vi "delete control from class private data.vi"(8 "error in":errorcluster, 9 "control label":string, 10 "path":path, 11 "Project in":refnum<vi>) -> (0 "error out":errorcluster, 3 "Project out":refnum<vi>)   [LabVIEW 2013, in "NISE Tools Scripting.lvlib"]
uses:
  NISE Tools Scripting.lvlib
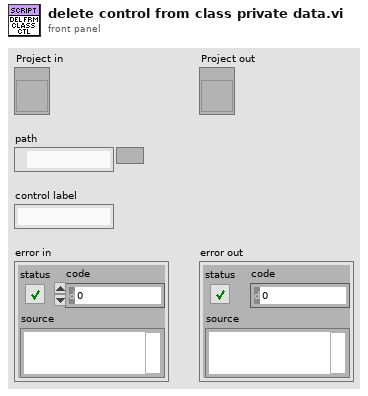
[diagram p1: front panel]
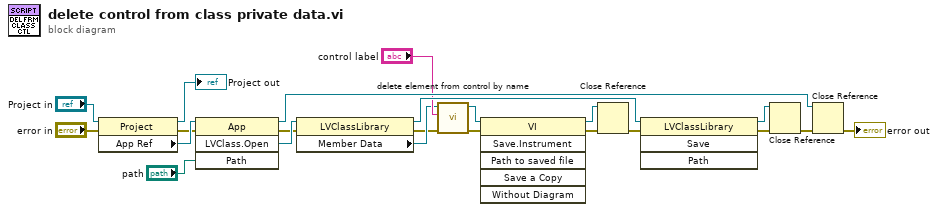
[diagram p0: block diagram]
diagram:
  n1 = property class="Project"(reference="Project in", error in="error in") -> (reference out=→"Project out":refnum<vi>, error out=w7:errorcluster, "App Ref"=w8:refnum<vi>)
  n2 = invoke class="App" method="LVClass.Open"(reference=w8, error in=w7, "Path"="path") -> (reference out=w18:refnum<vi>, error out=w10:errorcluster, "LVClass.Open"=w11:refnum<vi>)  [unwired: 1 in, 1 out]
  n3 = property class="LVClassLibrary"(reference=w11, error in=w10) -> (reference out=w17:refnum<vi>, error out=w12:errorcluster, "Member Data"=w13:refnum<vi>)
  n4 = call "delete element from control by name.vi"("error in"=w12, "control label"="control label", "VI in"=w13) -> ("error out"=w19:errorcluster, "reference out"=w3:refnum<vi>)  [unwired: 7 in]
  n5 = invoke class="VI" method="Save.Instrument"(reference=w3, error in=w19) -> (reference out=w1:refnum<vi>, error out=w4:errorcluster)  [unwired: 4 in, 4 out]
  n6 = Close Reference(reference=w1, error in (no error)=w4) -> (error out=w2:errorcluster)
  n7 = invoke class="LVClassLibrary" method="Save"(reference=w17, error in=w2) -> (reference out=w16:refnum<vi>, error out=w15:errorcluster)  [unwired: 2 in, 2 out]
  n8 = Close Reference(reference=w16, error in (no error)=w15) -> (error out=w20:errorcluster)
  n9 = Close Reference(reference=w18, error in (no error)=w20) -> (error out=→"error out":errorcluster)
